vi "Turret_Globals.vi"() -> ()   [LabVIEW 2019]
uses:
  Subsystems/Turret/Turret_Cluster.ctl
  Subsystems/Turret/Turret_States.ctl
panel:
  in  "Turret_Spin":string="Turret_Spin"
  in  "Turret_Execute_Notifier":refnum<notifier>
  in  "Turret_Set_Notifier":refnum<notifier>
  in  "Turret_Execute_Ref":string="Turret_Execute_Ref"
  in  "Turret_Set_Ref":string="Turret_Set_Ref"
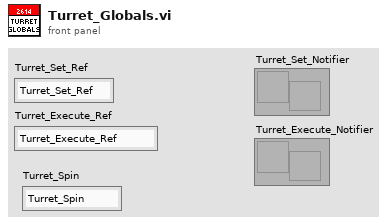
[diagram p1: front panel]
diagram:
